vi "gradient.vi"() -> ()   [LabVIEW 2020]
uses:
  <vilib>/Rock Robotics/SystemInterfaces/DIO/FPGA_DIOPWMChannel.ctl
  ArduinoSerialBling.lvlib
panel:
  in  "Color 2":u32(colorbox)=16860
  in  "Color 1":u32(colorbox)=16711680
  in  "Sine Rate":i32
  out "String Length":u16=144
  in  "PWM Channel":T1=enum."PWM 9"
  in  "stop":bool
  out "LED Strip":u32[](array[colorbox])
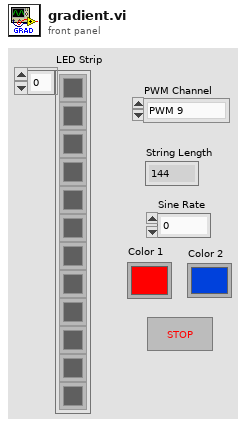
[diagram p1: front panel]
types:
  T1 = typedef "FPGA_DIOPWMChannel.ctl" = enum8{"PWM 0", "PWM 1", "PWM 2", "PWM 3", "PWM 4", "PWM 5", "PWM 6", "PWM 7", "PWM 8", "PWM 9", "PWM MXP 0", "PWM MXP 1", "PWM MXP 2", "PWM MXP 3", "PWM MXP 4", "PWM MXP 5", "PWM MXP 6", "PWM MXP 7", "PWM MXP 8", "PWM MXP 9", "Invalid"}
  T2 = typedef "WPI_PWMDeviceRef.ctl" = cluster{"DeviceStatus":errorcluster, "PWM Channel":T1}
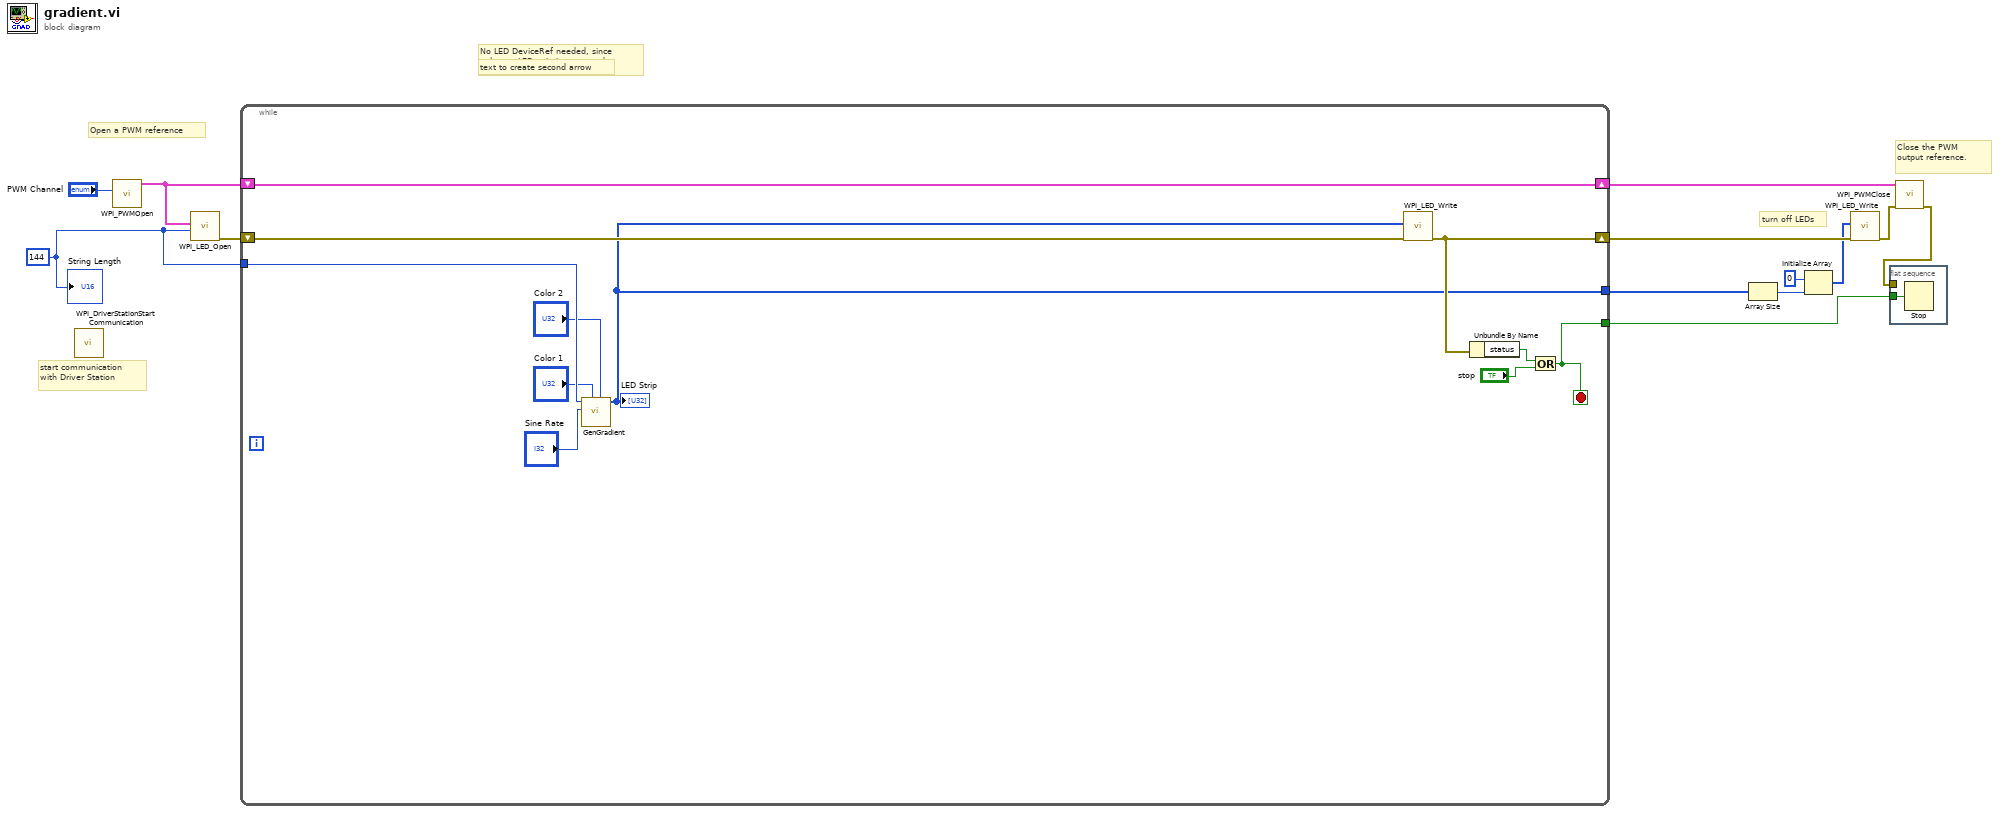
[diagram p0: block diagram]
diagram:
  w3 = u16 144 ("String Length")
  # "turn off LEDs"
  # "No LED DeviceRef needed, since only one LED strip is supported"
  # "Open a PWM reference"
  # "start communication with Driver Station"
  # "Close the PWM output reference."
  # "text to create second arrow"
  n1 = call <vilib>:"WPI_DriverStationStart Communication.vi"() -> ()  [unwired: 3 in, 9 out]
  n2 = call <vilib>:"WPI_PWMOpen.vi"("PWM Channel"="PWM Channel") -> ("PWMDeviceRef"=w11:T2)  [unwired: 9 in, 1 out]
  n3 = call <vilib>:"WPI_LED_Open.vi"("String Length"=w3, "PWMDeviceRef"=w11) -> ("error out"=w12:errorcluster)  [unwired: 9 in]
  n4 = while {
    shift-right: [w21] -> w13
    shift-left: w11 -> [w21]
    tunnel: [w24] -> w2
    shift-right: [w19] -> w9
    shift-left: w12 -> [w20]
    tunnel: w3 -> [w18]
    tunnel: [w17] -> w6
    stop <- w24 stop-if-true
    n5 = call "GenGradient.vi"("Color 2"="Color 2", "Color 1"="Color 1", "Sine Rate"="Sine Rate", "NumLeds"=w18) -> ("LED Array"=w17:u32[])  [unwired: 7 in]
    "LED Strip" <- w17
    n6 = call <vilib>:"WPI_LED_Write.vi"("error in"=w20, "Color Array"=w17) -> ("error out"=w19:errorcluster)  [unwired: 9 in]
    n7 = Unbundle By Name(w19) -> ("status"=w22:bool)
    n8 = Or(x=w22, y="stop") -> (x .or. y?=w24:bool)
  }
  n9 = Array Size(array=w6) -> (size(s)=w7:i32)
  n10 = Initialize Array(u32 0, w7) -> (w4:u32[])
  n11 = call <vilib>:"WPI_LED_Write.vi"("error in"=w9, "Color Array"=w4) -> ("error out"=w8:errorcluster)  [unwired: 9 in]
  n12 = flat-sequence {
    tunnel: w2 -> [w25]
    tunnel: w1 -> [_]
    frame #0 {
      n13 = Stop(stop? (T)=w25) -> ()
    }
  }
  n14 = call <vilib>:"WPI_PWMClose.vi"("error in (no error)"=w8, "PWMDeviceRef"=w13) -> ("error out"=w1:errorcluster)  [unwired: 9 in]
  "String Length" <- w3
